vi "pcfs_perform_pcfs.vi"(8 "error in (no error)":errorcluster, 11 "pcfs in":refnum<class "pcfs.lvclass">) -> (0 "error out":errorcluster, 3 "pcfs out":refnum<class "pcfs.lvclass">)   [LabVIEW 2015, in "pcfs.lvclass"]
uses:
  pcfs.lvclass
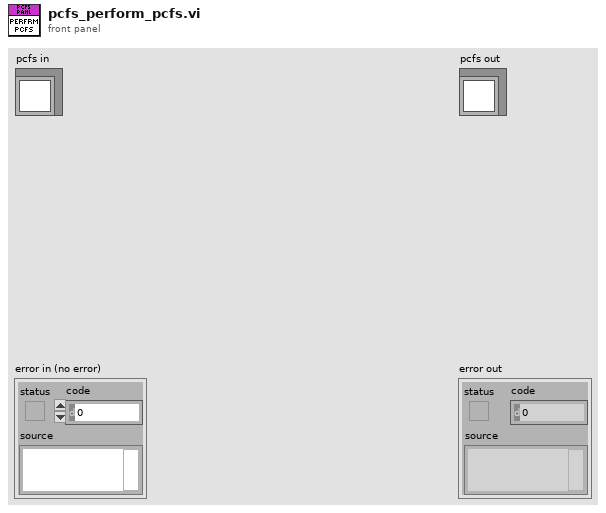
[diagram p1: front panel]
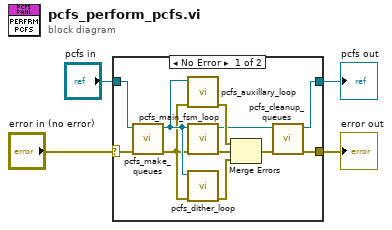
[diagram p0: block diagram]
diagram:
  n1 = case shown="No Error" "error in (no error)" {
    selector: "error in (no error)" -> [w9 w17]
    tunnel: [w7 w17] -> w3
    tunnel: [w5 w16] -> w1
    tunnel: "pcfs in" -> [w15 w16]
    frame No Error {
      n2 = call "pcfs_make_queues.vi"("error in (no error)"=w9, "pcfs in"=w15) -> ("error out"=w13:errorcluster, "pcfs out"=w14:refnum<class "pcfs.lvclass">)  [unwired: 8 in]
      n3 = call "pcfs_auxillary_loop.vi"("error in (no error)"=w13, "pcfs in"=w14) -> ("error out"=w12:errorcluster)  [unwired: 8 in, 1 out]
      n4 = call "pcfs_main_fsm_loop.vi"("error in (no error)"=w13, "pcfs in"=w14) -> ("error out"=w11:errorcluster, "pcfs out"=w6:refnum<class "pcfs.lvclass">)  [unwired: 8 in]
      n5 = call "pcfs_dither_loop.vi"("error in (no error)"=w13, "pcfs in"=w14) -> ("error out"=w10:errorcluster)  [unwired: 8 in, 1 out]
      n6 = Merge Errors(w12, w11, w10) -> (w8:errorcluster)
      n7 = call "pcfs_cleanup_queues.vi"("error in (no error)"=w8, "pcfs in"=w6) -> ("error out"=w7:errorcluster, "pcfs out"=w5:refnum<class "pcfs.lvclass">)  [unwired: 8 in]
    }
    frame Error {
    }
  }
  "error out" <- w3
  "pcfs out" <- w1
